vi "GetName.vi"(8 "error in (no error)":errorcluster, 11 "Animal in":refnum<class "Animal.lvclass">) -> (0 "error out":errorcluster, 2 "Name":string, 3 "Animal out":refnum<class "Animal.lvclass">)   [LabVIEW 2018, in "Animal.lvclass"]
uses:
  Animal.lvclass
  Animal.lvclass/Animal.ctl
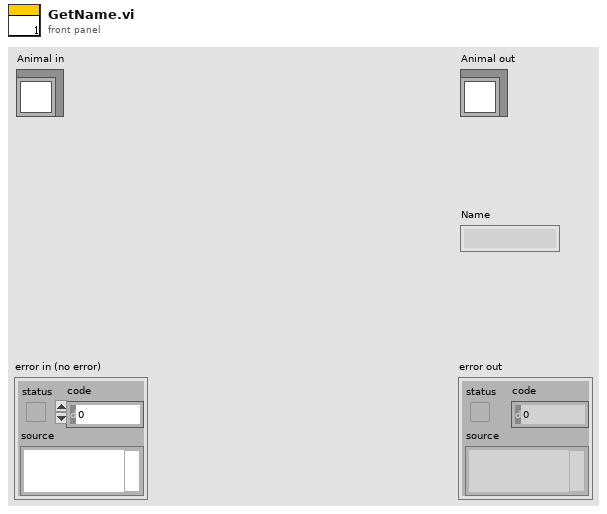
[diagram p1: front panel]
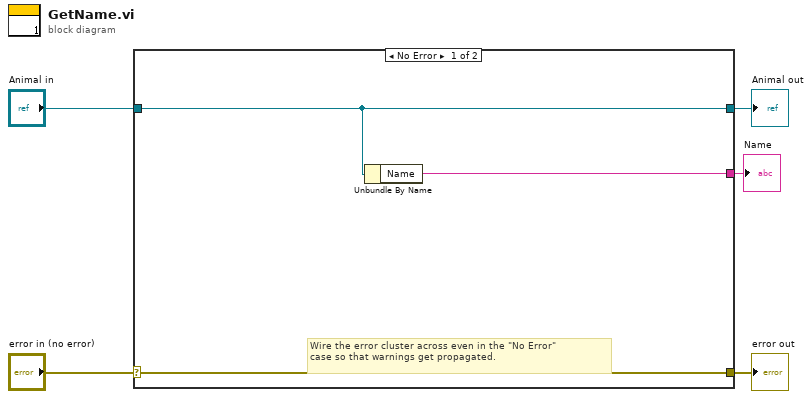
[diagram p0: block diagram]
diagram:
  n1 = case shown="No Error" "error in (no error)" {
    selector: "error in (no error)" -> [w8 w10]
    tunnel: [w8 w10] -> w4
    tunnel: [w7 w9] -> w2
    tunnel: "Animal in" -> [w7 w9]
    tunnel: [w6 _] -> w1
    frame No Error {
      # "Wire the error cluster across even in the \"No Error\"\ncase so that warnings get propagated."
      n2 = Unbundle By Name(w7) -> ("Name"=w6:string)
    }
    frame Error {
    }
  }
  "error out" <- w4
  "Animal out" <- w2
  "Name" <- w1
